vi "PositionToRollSkill.vi"(7 "Game in":refnum<class "Game.lvclass">, 8 "error in (no error)":errorcluster, 10 "Robot":refnum<class "Robot.lvclass">, 11 "PositionToRollSkill in":refnum<class "PositionToRollSkill.lvclass">) -> (0 "error out":errorcluster, 2 "Robot out":refnum<class "Robot.lvclass">, 3 "PositionToRollSkill out":refnum<class "PositionToRollSkill.lvclass">)   [LabVIEW 2020, in "PositionToRollSkill.lvclass"]
uses:
  PositionToRollSkill.lvclass
  Utilities_class/Utilities.lvclass
  Robot_class/roles.ctl
  Robot_class/Robot.lvclass
  C:/Users/Administrator/Desktop/SSL/SSL_AI/Object_class/Object.lvclass
  C:/Users/Administrator/Desktop/SSL/SSL_AI/Robot_class/Robot.lvclass
  Ball_class/Ball.lvclass
  Game_class/Game.lvclass
  Ally_class/Ally.lvclass
  C:/Users/Administrator/Desktop/SSL/SSL_AI/Ball_class/Ball.lvclass
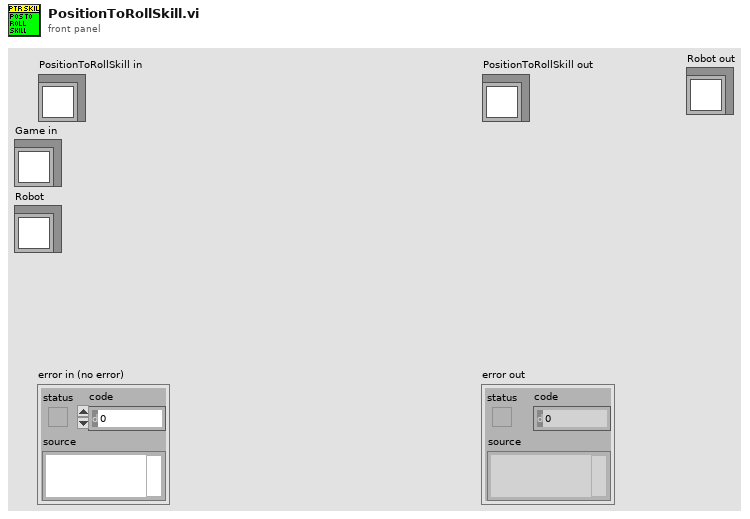
[diagram p1: front panel]
types:
  T1 = typedef "roles.ctl" = enum16{"PreparePassReceiver 3", "SecondMarker", "WaitPass", "ABCThirdKicker", "ABCFirstKicker", "ABCSecondKicker", "Tabler", "TableFinalizer", "PrepareRollToPassRoller", "PrepareRollToPassReceiver", "SimplePassRoll", "SimplePassRollReceiver", "PenaltyDefense", "PreparePassReceiver 2", "PreparePassReceiver 1", "PassObserver", "Timeout", "Goto", "ZigZag", "None", "BallOutOfField", "DefenderArea", "Duelist", "AttackerStop", "FollowAttacker", "KeeperRole", "KickPenalty", "AttackerAimGoal", "AttackerBlock", "Marker", "Halt", "Shoot", "PassKicker", "PassReceiver", "TestRole", "PenaltyAttacker"}
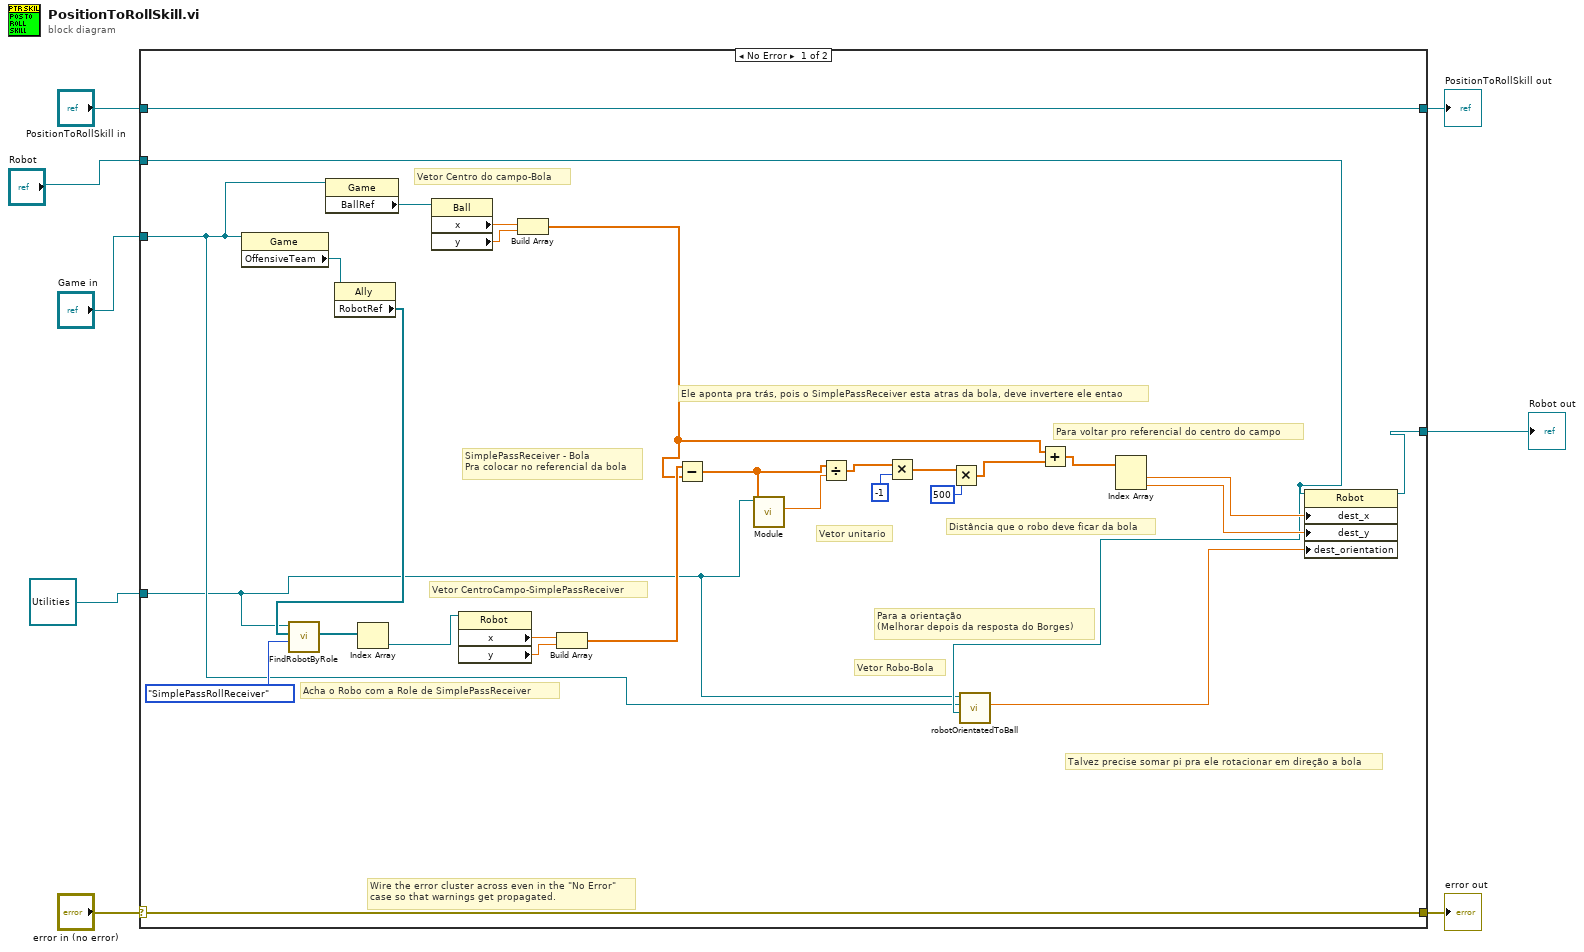
[diagram p0: block diagram]
diagram:
  n1 = case shown="No Error" "error in (no error)" {
    selector: "error in (no error)" -> [w36 w40]
    tunnel: [w36 w40] -> w7
    tunnel: [w37 w39] -> w5
    tunnel: "PositionToRollSkill in" -> [w37 w39]
    tunnel: "Game in" -> [w11 _]
    tunnel: refnum<class "Utilities.lvclass"> refnum ("Utilities in") -> [w10 _]
    tunnel: "Robot" -> [w12 w38]
    tunnel: [w16 w38] -> w1
    frame No Error {
      # "Talvez precise somar pi pra ele rotacionar em direção a bola"
      # "Vetor Robo-Bola"
      # "Para a orientação\n(Melhorar depois da resposta do Borges)"
      # "Para voltar pro referencial do centro do campo"
      # "Distância que o robo deve ficar da bola"
      # "Ele aponta pra trás, pois o SimplePassReceiver esta atras da bola, deve invertere ele entao"
      # "Vetor unitario"
      # "SimplePassReceiver - Bola\nPra colocar no referencial da bola"
      # "Vetor CentroCampo-SimplePassReceiver"
      # "Vetor Centro do campo-Bola"
      # "Acha o Robo com a Role de SimplePassReceiver"
      # "Wire the error cluster across even in the \"No Error\"\ncase so that warnings get propagated."
      n2 = property class="Game"(reference=w11) -> ("OffensiveTeam"=w35:refnum<class "Ally.lvclass">)  [unwired: 1 in, 2 out]
      n3 = property class="Game"(reference=w11) -> ("BallRef"=w30:refnum<class "Ball.lvclass">)  [unwired: 1 in, 2 out]
      n4 = property class="Ally"(reference=w35) -> ("RobotRef"=w34:refnum<class "Robot.lvclass">[])  [unwired: 1 in, 2 out]
      n5 = call "FindRobotByRole.vi"("role"=roles."SimplePassRollReceiver", "RobotRef"=w34, "Utilities in"=w10) -> ("Robots"=w32:refnum<class "Robot.lvclass">[])  [unwired: 6 in, 2 out]
      n6 = Index Array(array=w32) -> (element=w31:refnum<class "Robot.lvclass">)  [unwired: 1 in]
      n7 = property class="Ball"(reference=w30) -> ("x"=w29:dbl, "y"=w28:dbl)  [unwired: 1 in, 2 out]
      n8 = property class="Robot"(reference=w31) -> ("x"=w27:dbl, "y"=w26:dbl)  [unwired: 1 in, 2 out]
      n9 = Build Array(w29, w28) -> (w14:dbl[])
      n10 = Build Array(w27, w26) -> (w23:dbl[])
      n11 = Subtract(x=w23, y=w14) -> (x-y=w25:dbl[])
      n12 = call-dynamic "Module.vi"("2D vector"=w25, "Utilities in"=w10) -> ("Modulo"=w24:dbl)  [unwired: 7 in, 2 out]
      n13 = Divide(x=w25, y=w24) -> (x/y=w22:dbl[])
      n14 = Multiply(x=w22, y=-1) -> (x*y=w20:dbl[])
      n15 = Multiply(x=w20, y=500) -> (x*y=w13:dbl[])
      n16 = call "robotOrientatedToBall.vi"("Robot"=w12, "BallRef"=w11, "Utilities in"=w10) -> ("Orientation"=w9:dbl)  [unwired: 6 in, 2 out]
      n17 = Add(x=w14, y=w13) -> (x+y=w15:dbl[])
      n18 = Index Array(array=w15) -> (element #1=w18:dbl, element #2=w17:dbl)  [unwired: 2 in]
      n19 = property class="Robot"(reference=w12, "dest_x"=w18, "dest_y"=w17, "dest_orientation"=w9) -> (reference out=w16:refnum<class "Robot.lvclass">)  [unwired: 1 in, 1 out]
    }
    frame Error {
    }
  }
  "error out" <- w7
  "PositionToRollSkill out" <- w5
  "Robot out" <- w1
